vi "SPI Read Register.vi"(6 "Register":u8, 7 "CS Pin":i32, 8 "error in (no error)":errorcluster, 9 "Len":u8, 10 "Bus":u8, 11 "VISA resource name in":refnum<visa-resource-name>) -> (0 "error out":errorcluster, 1 "Data":string, 3 "VISA resource name":refnum<visa-resource-name>)   [LabVIEW 2023, in "CTI-Visa-DeviceLib.lvlib"]
uses:
  CTI-Visa-DeviceLib.lvlib
  de3d6c1a-80d7-4754-9d99-d16a6bf6a74c.vi
  CTI-Visa/CTI-Visa.lvlib
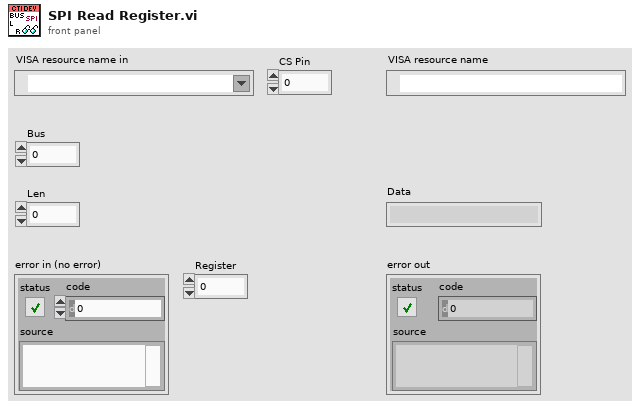
[diagram p1: front panel]
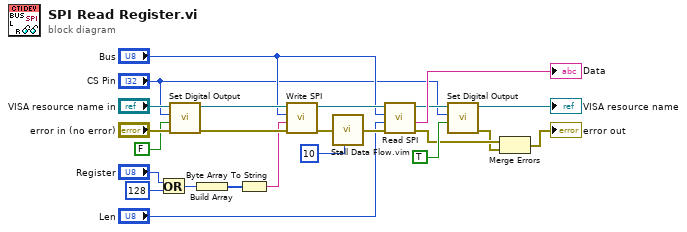
[diagram p0: block diagram]
diagram:
  n1 = Or(x="Register", y=u8 128) -> (x .or. y?=w17:u8)
  n2 = call "Set Digital Output.vi"("error in (no error)"="error in (no error)", "Value"=FALSE, "Channel"="CS Pin", "VISA resource name in"="VISA resource name in") -> ("error out"=w18:errorcluster, "VISA resource name"=w19:refnum<visa-resource-name>)  [unwired: 6 in]
  n3 = Build Array(w17) -> (w16:u8[])
  n4 = Byte Array To String(unsigned byte array=w16) -> (string=w15:string)
  n5 = call "Write SPI.vi"("error in (no error)"=w18, "Data"=w15, "Bus"="Bus", "VISA resource name in"=w19) -> ("error out"=w14:errorcluster, "VISA resource name"=w11:refnum<visa-resource-name>)  [unwired: 6 in]
  n6 = call "Stall Data Flow.vim"("value in"=w14, "milliseconds to wait"=u32 10) -> ("value out"=w12:errorcluster)  [unwired: 1 out]
  n7 = call "Read SPI.vi"("error in (no error)"=w12, "Len"="Len", "Bus"="Bus", "VISA resource name in"=w11) -> ("error out"=w3:errorcluster, "Data"=→"Data":string, "VISA resource name"=w7:refnum<visa-resource-name>)  [unwired: 5 in]
  n8 = call "Set Digital Output.vi"("Value"=TRUE, "Channel"="CS Pin", "VISA resource name in"=w7) -> ("error out"=w2:errorcluster, "VISA resource name"=→"VISA resource name":refnum<visa-resource-name>)  [unwired: 7 in]
  n9 = Merge Errors(w3, w2) -> (→"error out":errorcluster)
